vi "Post Substeps Analog Input Task.vi"(9 "Socket No":u16=1, 10 "AIRead":T1, 11 "Sequence Context In":refnum<k7>) -> (0 "error out":errorcluster, 1 "Selected Physical Channel":string[](array[string]), 2 "AnalogRead":dbl[](array[numeric]), 3 "Report Text":string)   [LabVIEW 2023, in "LTT_TeststandSteptypes.lvlib"]
doc: "This VI is Anaload Input Read MultiNumeric Test and PostSub Steptypes"
uses:
  LTT_TeststandSteptypes.lvlib
  HardwareAbstractionLayer_LVOOP/Main/Class Options.ctl
  HardwareAbstractionLayer_LVOOP/Analog Input/AI/AI.lvclass
  HardwareAbstractionLayer_LVOOP/Main/Main.lvclass
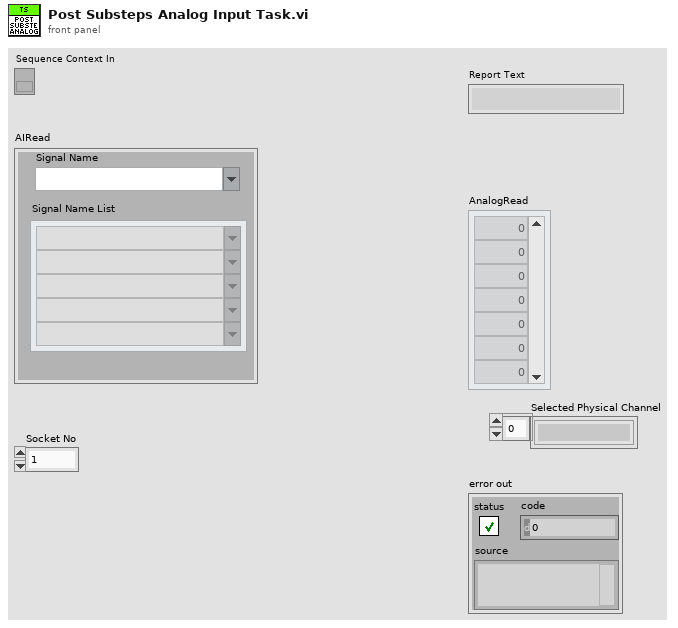
[diagram p1: front panel]
types:
  T1 = cluster{"Signal Name":string, "Signal Name List":string[]}
  T2 = typedef "HardwareAbstractionLayer_LVOOP.lvlib/Main.lvclass/Class Options.ctl" = enum16{"Init All Class", "Read All Class", "Write AI Class", "Write AO Class", "Write AO Waveform Generation", "Write DI Class", "Write DO Class", "Write PWM Input Class", "Write PWM Output Class", "Exit"}
  T3 = typedef "HardwareAbstractionLayer_LVOOP.lvlib/Main.lvclass/Class Ref.ctl" = cluster{"FGV":refnum<class "Function Global Variable.lvclass">, "Notifier":refnum<class "NotifierHandler.lvclass">, "Queue":refnum<class "Queue Handler.lvclass">, "User Event":refnum<class "User Event.lvclass">, "Data Manager":refnum<class "Data Manager.lvclass">, "DMM":refnum<class "DMM.lvclass">, "Function Generator":refnum<class "Function Generator.lvclass">, "Oscilloscope":refnum<class "Oscilloscope.lvclass">, "PowerSupply":refnum<class "PowerSupply.lvclass">, "Teststand":refnum<class "Teststand.lvclass">, "AO":refnum<class "AO.lvclass">, "AI":refnum<class "AI.lvclass">, "Database":refnum<class "Database.lvclass">, "AO Waveform Generation":refnum<class "AO.lvclass">, "DO":refnum<class "DO.lvclass">, "DI":refnum<class "DI.lvclass">, "PWM Output":refnum<class "PWM Output.lvclass">, "PWM Input":refnum<class "PWM Input.lvclass">, "RelayOutput":refnum<class "NISwitch.lvclass">, "Modbus":refnum<class "Modbus.lvclass">, "CAN":refnum<class "CAN.lvclass">}
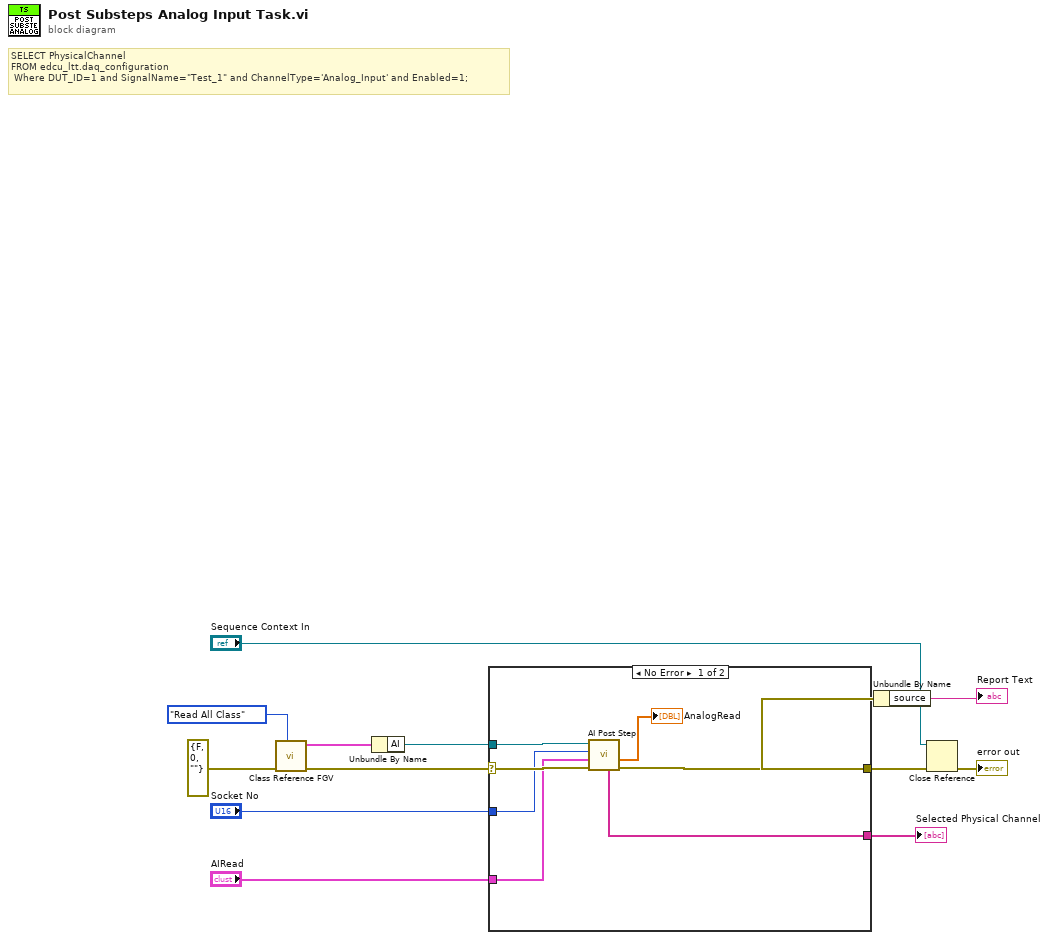
[diagram p0: block diagram]
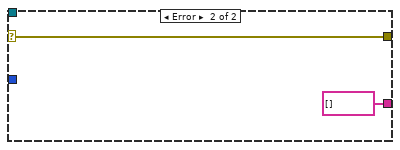
[diagram p2: hidden frame]
diagram:
  # "SELECT PhysicalChannel \nFROM edcu_ltt.daq_configuration\n Where DUT_ID=1 and SignalName=\"Test_1\" and ChannelType='Analog_Input' and Enabled=1;"
  n1 = call "Class Reference FGV.vi"("Options"=Class_Options."Read All Class", "error in"=errorcluster {"status"=FALSE, "code"=0, "source"=""}) -> ("error out"=w7:errorcluster, "Class Cluster Out"=w9:T3)  [unwired: 8 in]
  n2 = Unbundle By Name(w9) -> ("AI"=w6:refnum<class "AI.lvclass">)
  n3 = case shown="No Error" w7 {
    selector: w7 -> [w18 w21]
    tunnel: w6 -> [w19 _]
    tunnel: [w17 w21] -> w5
    tunnel: "Socket No" -> [w15 _]
    tunnel: "AIRead" -> [w14 _]
    tunnel: [w13 string[] [] ("Selected Physical Channel")] -> w1
    frame No Error {
      n4 = call-dynamic "AI Post Step.vi"("error in (no error)"=w18, "AIRead"=w14, "Socket No"=w15, "AI in"=w19) -> ("error out"=w17:errorcluster, "AnalogRead"=→"AnalogRead":dbl[], "Selected Physical Channel"=w13:string[])  [unwired: 3 in, 2 out]
    }
    frame Error {
    }
  }
  "Selected Physical Channel" <- w1
  n5 = Unbundle By Name(w5) -> ("source"=→"Report Text":string)
  n6 = Close Reference(reference="Sequence Context In", error in (no error)=w5) -> (error out=→"error out":errorcluster)
